vi "SetIMMode.vi"(6 "Legacy (f)?":bool, 8 "error in (no error)":errorcluster, 10 "SetIMMode":T1 items=["Reverse", "Forward", "Auxiliary"]) -> (0 "error out":errorcluster)   [LabVIEW 2011]
uses:
  MeasMode.ctl
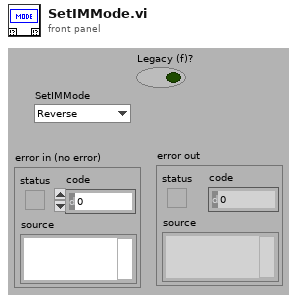
[diagram p1: front panel]
types:
  T1 = typedef "MeasMode.ctl" = u16
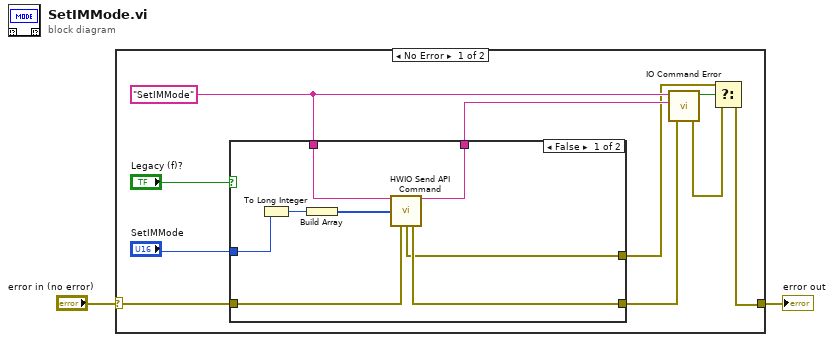
[diagram p0: block diagram]
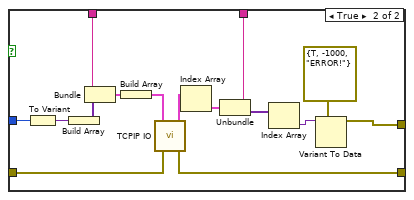
[diagram p2: hidden frame]
diagram:
  n1 = case shown="No Error" "error in (no error)" {
    selector: "error in (no error)" -> [w8 w36]
    tunnel: [w4 w36] -> w2
    frame No Error {
      w10 = "SetIMMode"
      n2 = case shown="False" "Legacy (f)?" {
        tunnel: "SetIMMode" -> [w16 w33]
        tunnel: [w18 w30] -> w11
        tunnel: w10 -> [w17 w29]
        tunnel: [w19 w28] -> w9
        tunnel: w8 -> [w20 w25]
        tunnel: [w13 w22] -> w7
        frame False {
          n3 = To Long Integer(number=w16) -> (32bit integer=w15:i32)
          n4 = Build Array(w15) -> (w14:i32[])
          n5 = call "HWIO Send API Command.vi"("Action"=w17, "Integer"=w14, "error in (no error)"=w20) -> ("Action out"=w18:string, "HWError"=w13:errorcluster, "error out"=w19:errorcluster)  [unwired: 5 in, 5 out]
        }
        frame True {
          n6 = To Variant(anything=w33) -> (Variant=w35:variant)
          n7 = Build Array(w35) -> (w34:variant[])
          n8 = Bundle(w29, w34) -> (w31:cluster{string, variant[]})  [unwired: 1 out]
          n9 = Build Array(w31) -> (w32:cluster{string, variant[]}[])
          n10 = call "TCPIP IO.vi"("error in (no error)"=w25, "Commands"=w32) -> ("error out"=w28:errorcluster, "Responses"=w26:cluster{string, variant[]}[])  [unwired: 1 in, 3 out]
          n11 = Index Array(array=w26) -> (element=w27:cluster{string, variant[]})  [unwired: 1 in]
          n12 = Unbundle(w27) -> (w30:string, w21:variant[])
          n13 = Index Array(array=w21) -> (element=w24:variant)  [unwired: 1 in]
          n14 = Variant To Data(type=errorcluster {"status"=TRUE, "code"=-1000, "source"="ERROR!"} ("error out"), Variant=w24) -> (data=w22:errorcluster)  [unwired: 1 in, 1 out]
        }
      }
      n15 = call "IO Command Error.vi"("error in (no error)"=w9, "Command Returned (\"\")"=w11, "Command Sent (\"\")"=w10) -> ("error out"=w5:errorcluster, "HW ERR?"=w6:bool)  [unwired: 3 out]
      n16 = Select(t=w7, s=w6, f=w5) -> (s? t:f=w4:errorcluster)
    }
    frame Error {
    }
  }
  "error out" <- w2
